vi "Main.vi"(8 "error in (no error)":errorcluster, 11 "Demo App in":refnum<class "Demo App.lvclass">) -> (0 "error out":errorcluster, 3 "Demo App out":refnum<class "Demo App.lvclass">)   [LabVIEW 2018, in "Demo App.lvclass"]
uses:
  Demo App.lvclass
  ConsoleOut/Print Options.ctl
  Product Class/ProductA_Factory.lvclass
  C:/Users/fflores/Documents/LabVIEW-Open-Projects/LabIVEW OOP Design Patterns/Factory Method Pattern/Factory Class/Factory.lvclass
  Factory Class/ProductB_Factory/ProductB_Factory.lvclass
  Factory Class/Factory.lvclass
  Product Class/Product/Product.lvclass
panel:
  in  "Choose Product":enum16{"Product A", "Product B"}(ring)
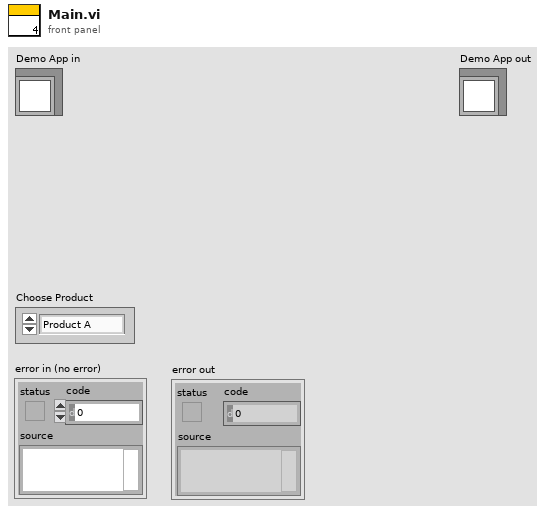
[diagram p1: front panel]
types:
  T1 = typedef "Print Options.ctl" = enum16{"Create", "Get Reference", "Print", "Print Header", "Close"}
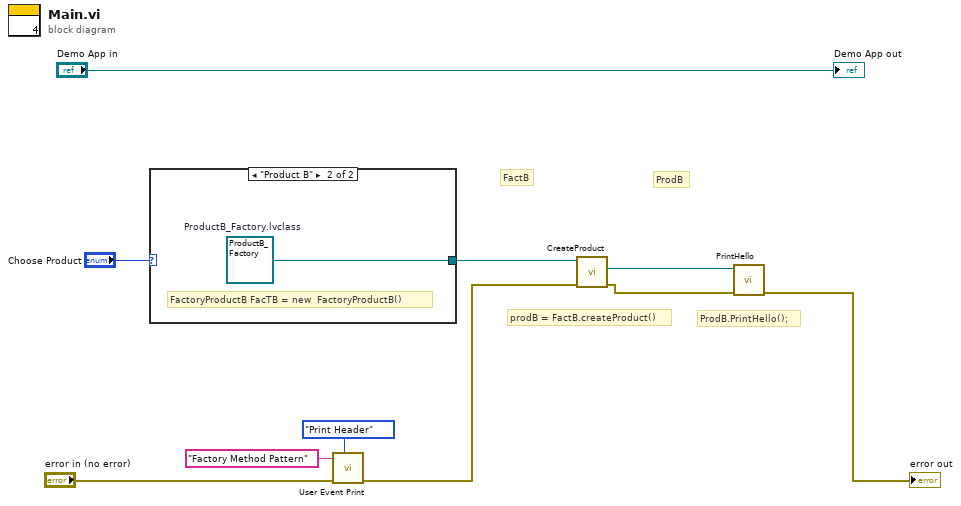
[diagram p0: block diagram]
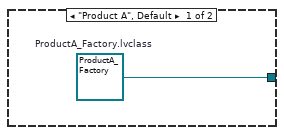
[diagram p2: hidden frame]
diagram:
  # "ProdB.PrintHello();"
  # "ProdB"
  # "FactB"
  # "prodB = FactB.createProduct()"
  n1 = case shown="\"Product B\"" "Choose Product" {
    tunnel: [w11 w12] -> w8
    frame "Product A", Default {
      w11 = refnum<class "ProductA_Factory.lvclass"> refnum  # ProductA_Factory.lvclass
    }
    frame "Product B" {
      w12 = refnum<class "ProductB_Factory.lvclass"> refnum  # ProductB_Factory.lvclass
      # "FactoryProductB FacTB = new  FactoryProductB()"
    }
  }
  n2 = call "User Event Print.vi"("Options"=Print_Options."Print Header", "error in (no error)"="error in (no error)", "String to Print"="Factory Method Pattern") -> ("error out"=w2:errorcluster)  [unwired: 7 in, 1 out]
  n3 = call-dynamic "CreateProduct.vi"("error in (no error)"=w2, "Factory in"=w8) -> ("error out"=w3:errorcluster, "Product.lvclass"=w7:refnum<class "Product.lvclass">)  [unwired: 7 in, 1 out]
  n4 = call-dynamic "PrintHello.vi"("error in (no error)"=w3, "Product in"=w7) -> ("error out"=→"error out":errorcluster)  [unwired: 8 in, 1 out]
  "Demo App out" <- "Demo App in"
